vi "testNoError.vi"() -> ()   [LabVIEW 2019, in "AssertionTest.lvlib" / "AssertErrorCode.lvlib"]
uses:
  AssertErrorCode.lvlib
  c1be48e0-8893-4c09-ba40-1e86d22c716c.vi
  Constraint/IsEqual/Create.vi
  Constraint/IsEqual/IsEqual.lvclass
  Assertion/Assertion.lvlib
panel:
  out "error out":errorcluster
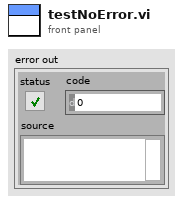
[diagram p1: front panel]
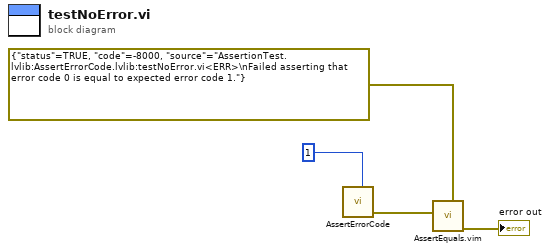
[diagram p0: block diagram]
diagram:
  n1 = call "AssertErrorCode.vi"("Expected"=1) -> ("error out"=w3:errorcluster)  [unwired: 10 in]
  n2 = call "AssertEquals.vim"("Expected"=errorcluster {"status"=TRUE, "code"=-8000, "source"="AssertionTest.lvlib:AssertErrorCode.lvlib:testNoError.vi<ERR>\nFailed asserting that error code 0 is equal to expected error code 1."} ("error out 2"), "Actual"=w3) -> ("error out"=→"error out":errorcluster)  [unwired: 9 in]
